vi "Scalar FPGA Personality.vi"() -> ()   [LabVIEW 2018]
uses:
  cRIO RT/TypeDefs/Simple cluster.ctl
  cRIO RT/TypeDefs/Complex cluster.ctl
  <vilib>/rvi/Emulation/niFpgaGetClockAttributes.vi
  <vilib>/rvi/Emulation/niFpgaSctlEmulationGetInTimedLoop.vi
  <vilib>/rvi/Emulation/niFpgaEmulationReportErrorSimple.vi
  <vilib>/rvi/Emulation/niFpgaCriticalErrorInLSC.vi
panel:
  out "Numeric FXP 23/23 out":fxp<+,23,23>
  in  "Numeric FXP 23/23 in":fxp<+,23,23>
  out "Numeric FXP 64/12 out":fxp<+/-,64,12>
  in  "Numeric FXP 64/12 in":fxp<+/-,7,3>
  out "Numeric FXP 7/3 out":fxp<+/-,7,3>
  in  "Numeric FXP 7/3 in":fxp<+/-,64,12>
  in  "Boolean in":bool
  out "Complex cluster out":T1
  in  "Complex cluster in":T1
  out "Simple cluster out":T2
  in  "Simple cluster in":T2
  in  "Numeric FXP 32/16 in":fxp<+/-,32,16>
  in  "Numeric U8 in":u8
  in  "Numeric U16 in":u16
  in  "Numeric U32 in":u32
  in  "Numeric U64 in":u64
  in  "Numeric I8 in":i8
  in  "Numeric I32 in":i32
  in  "Numeric I64 in":i64
  in  "Numeric SGL in":sgl
  in  "Numeric I16 in":i16
  out "Boolean out":bool
  out "Numeric U8 out":u8
  out "Numeric U16 out":u16
  out "Numeric U32 out":u32
  out "Numeric U64 out":u64
  out "Numeric I8 out":i8
  out "Numeric I32 out":i32
  out "Numeric I64 out":i64
  out "Numeric FXP 32/16 out":fxp<+/-,32,16>
  out "Numeric SGL out":sgl
  out "Numeric I16 out":i16
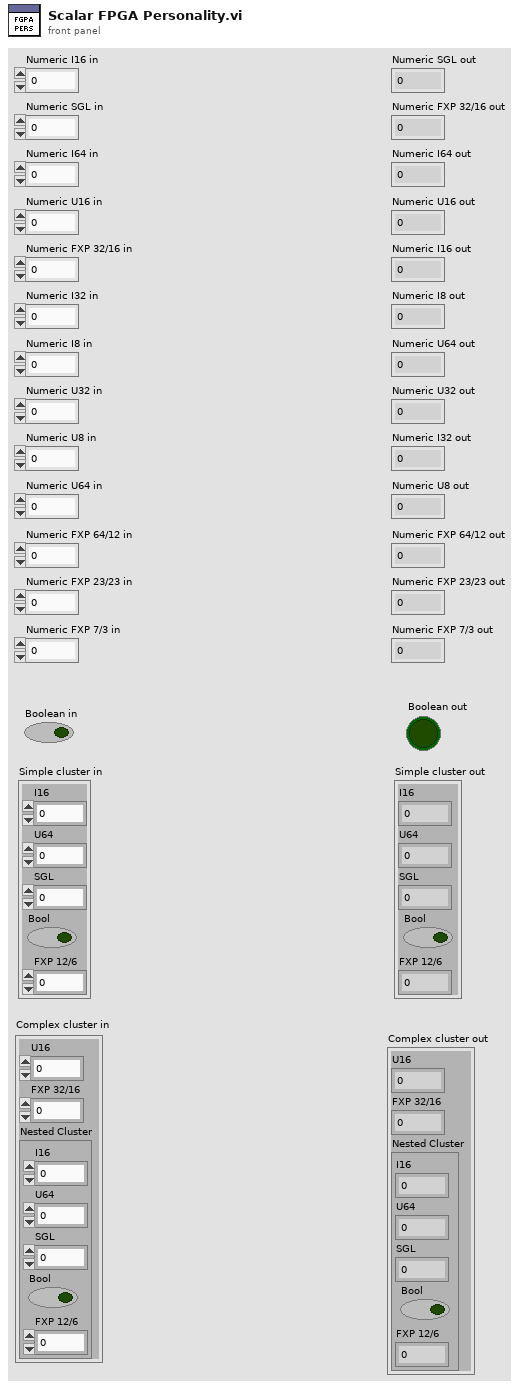
[diagram p1: front panel]
types:
  T1 = typedef "Complex cluster.ctl" = cluster{"U16":u16, "FXP 32/16":fxp<+/-,32,16>, "Nested Cluster":T2}
  T2 = typedef "Simple cluster.ctl" = cluster{"I16":i16, "U64":u64, "SGL":sgl, "Bool":bool, "FXP 12/6":fxp<+/-,12,6>}
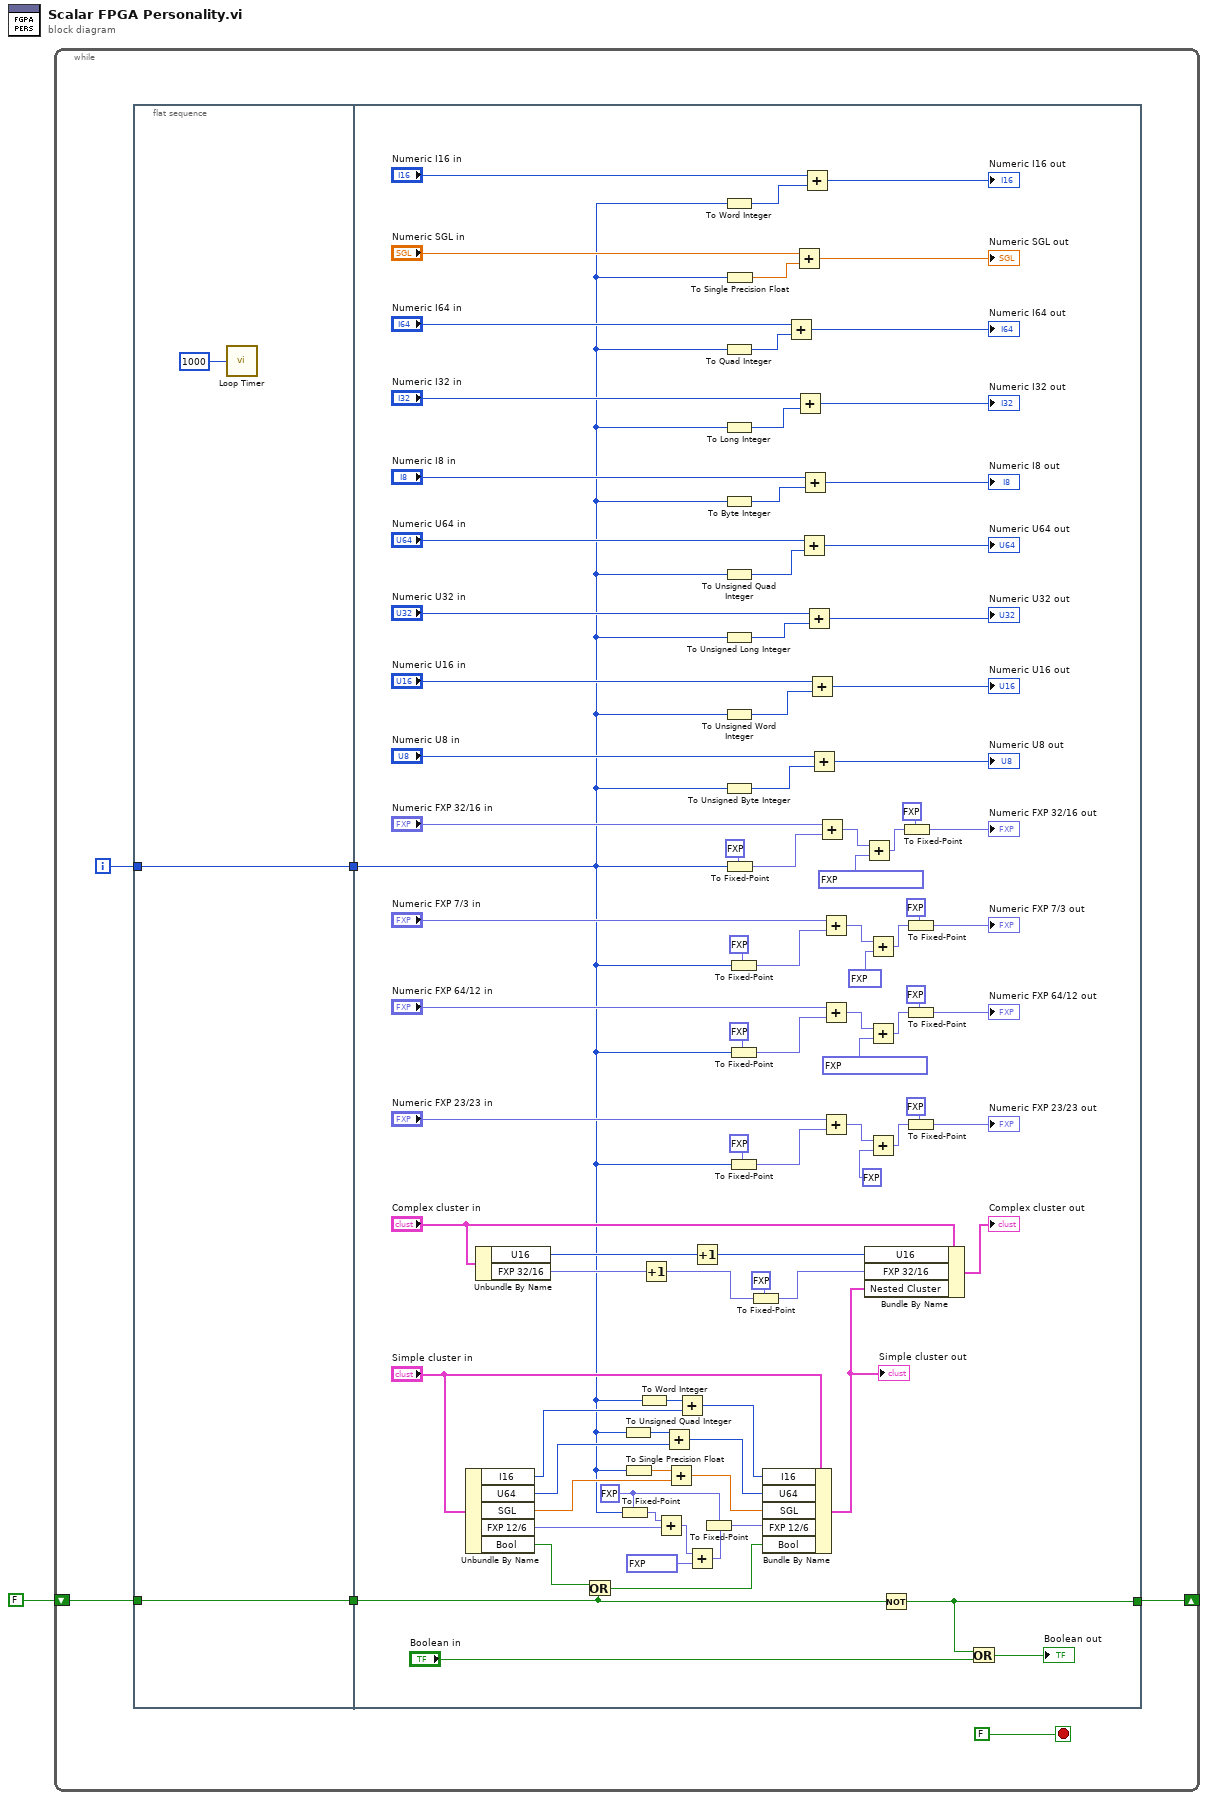
[diagram p0: block diagram]
diagram:
  n1 = while {
    shift-right: [w2] -> _
    shift-left: FALSE -> [w4]
    i -> [w6]
    stop <- FALSE stop-if-true
    n2 = flat-sequence {
      tunnel: w6 -> [w9]
      tunnel: [w9] -> w5
      tunnel: w4 -> [w8]
      tunnel: [w8] -> w3
      tunnel: w5 -> [w11]
      tunnel: w3 -> [w60]
      tunnel: [w38] -> w2
      frame #0 {
        n3 = call "Loop Timer"("Count(mSec)"=u32 1000) -> ()  [unwired: 1 out]
      }
      frame #1 {
        w43 = fxp<+/-,12,6> 0.0 ("FXP 12/6")
        n4 = Unbundle By Name("Simple cluster in") -> ("I16"=w70:i16, "U64"=w69:u64, "SGL"=w65:sgl, "FXP 12/6"=w62:fxp<+/-,12,6>, "Bool"=w59:bool)
        n5 = Unbundle By Name("Complex cluster in") -> ("U16"=w54:u16, "FXP 32/16"=w52:fxp<+/-,32,16>)
        n6 = Or(x=w59, y=w60) -> (x .or. y?=w58:bool)
        n7 = To Fixed-Point(fixed-point type=w43, number=w11) -> (fixed-point=w61:fxp<+/-,12,6>)
        n8 = To Unsigned Quad Integer(1:w11) -> (0:w68:u64)
        n9 = To Single Precision Float(number=w11) -> (single precision float=w64:sgl)
        n10 = To Word Integer(number=w11) -> (16bit integer=w71:i16)
        n11 = Increment(x=w52) -> (x+1=w45:fxp<+/-,33,17>)
        n12 = Add(x=w61, y=w62) -> (x+y=w41:fxp<+/-,13,7>)
        n13 = Add(x=w68, y=w69) -> (x+y=w66:u64)
        n14 = Add(x=w64, y=w65) -> (x+y=w63:sgl)
        n15 = Add(x=w71, y=w70) -> (x+y=w67:i16)
        n16 = Add(x=w41, y=fxp<+/-,12,6> 0.109375 ("FXP 12/6")) -> (x+y=w40:fxp<+/-,14,8>)
        n17 = Increment(x=w54) -> (x+1=w53:u16)
        n18 = To Fixed-Point(fixed-point type=w43, number=w40) -> (fixed-point=w42:fxp<+/-,12,6>)
        n19 = To Word Integer(number=w11) -> (16bit integer=w101:i16)
        n20 = To Quad Integer(1:w11) -> (0:w95:i64)
        n21 = To Long Integer(number=w11) -> (32bit integer=w92:i32)
        n22 = To Byte Integer(number=w11) -> (8bit integer=w89:i8)
        n23 = To Unsigned Quad Integer(1:w11) -> (0:w86:u64)
        n24 = To Unsigned Long Integer(number=w11) -> (unsigned 32bit integer=w83:u32)
        n25 = To Unsigned Word Integer(number=w11) -> (unsigned 16bit integer=w80:u16)
        n26 = To Unsigned Byte Integer(number=w11) -> (unsigned 8bit integer=w77:u8)
        n27 = To Single Precision Float(number=w11) -> (single precision float=w98:sgl)
        n28 = To Fixed-Point(fixed-point type=fxp<+/-,32,16> 0.0, number=w11) -> (fixed-point=w74:fxp<+/-,32,16>)
        n29 = To Fixed-Point(fixed-point type=fxp<+/-,64,12> 0.0, number=w11) -> (fixed-point=w29:fxp<+/-,64,12>)
        n30 = To Fixed-Point(fixed-point type=fxp<+/-,64,12> 0.0, number=w11) -> (fixed-point=w26:fxp<+/-,64,12>)
        n31 = To Fixed-Point(fixed-point type=fxp<+,23,23> 0.0, number=w11) -> (fixed-point=w13:fxp<+,23,23>)
        n32 = To Fixed-Point(fixed-point type=fxp<+/-,32,16> 0.0, number=w45) -> (fixed-point=w44:fxp<+/-,32,16>)
        n33 = Bundle By Name(cluster="Simple cluster in", "I16"=w67, "U64"=w66, "SGL"=w63, "FXP 12/6"=w42, "Bool"=w58) -> (w57:T2)
        "Simple cluster out" <- w57
        n34 = Add(x="Numeric I64 in", y=w95) -> (x+y=→"Numeric I64 out":i64)
        n35 = Add(x="Numeric SGL in", y=w98) -> (x+y=→"Numeric SGL out":sgl)
        n36 = Add(x="Numeric I32 in", y=w92) -> (x+y=→"Numeric I32 out":i32)
        n37 = Add(x="Numeric U64 in", y=w86) -> (x+y=→"Numeric U64 out":u64)
        n38 = Add(x="Numeric I8 in", y=w89) -> (x+y=→"Numeric I8 out":i8)
        n39 = Add(x="Numeric I16 in", y=w101) -> (x+y=→"Numeric I16 out":i16)
        n40 = Add(x="Numeric U32 in", y=w83) -> (x+y=→"Numeric U32 out":u32)
        n41 = Add(x="Numeric U16 in", y=w80) -> (x+y=→"Numeric U16 out":u16)
        n42 = Add(x="Numeric U8 in", y=w77) -> (x+y=→"Numeric U8 out":u8)
        n43 = Add(x="Numeric FXP 32/16 in", y=w74) -> (x+y=w49:fxp<+/-,33,17>)
        n44 = Add(x="Numeric FXP 7/3 in", y=w29) -> (x+y=w33:fxp<+/-,64,13>)
        n45 = Add(x="Numeric FXP 64/12 in", y=w26) -> (x+y=w22:fxp<+/-,64,13>)
        n46 = Add(x="Numeric FXP 23/23 in", y=w13) -> (x+y=w17:fxp<+,24,24>)
        n47 = Add(x=w49, y=fxp<+/-,33,17> 0.111114501953125) -> (x+y=w48:fxp<+/-,34,18>)
        n48 = Bundle By Name(cluster="Complex cluster in", "U16"=w53, "FXP 32/16"=w44, "Nested Cluster"=w57) -> (→"Complex cluster out":T1)
        n49 = Add(x=w33, y=fxp<+/-,7,3> 0.125) -> (x+y=w34:fxp<+/-,64,14>)
        n50 = Add(x=w22, y=fxp<+/-,64,12> 0.111114501953125) -> (x+y=w21:fxp<+/-,64,14>)
        n51 = Add(x=w17, y=fxp<+,23,23> 0.0) -> (x+y=w18:fxp<+,25,25>)
        n52 = Not(x=w60) -> (.not. x?=w38:bool)
        n53 = To Fixed-Point(fixed-point type=fxp<+/-,32,16> 0.0, number=w48) -> (fixed-point=→"Numeric FXP 32/16 out":fxp<+/-,32,16>)
        n54 = To Fixed-Point(fixed-point type=fxp<+/-,7,3> 0.0, number=w34) -> (fixed-point=→"Numeric FXP 7/3 out":fxp<+/-,7,3>)
        n55 = To Fixed-Point(fixed-point type=fxp<+/-,64,12> 0.0, number=w21) -> (fixed-point=→"Numeric FXP 64/12 out":fxp<+/-,64,12>)
        n56 = To Fixed-Point(fixed-point type=fxp<+/-,23,23> 0.0, number=w18) -> (fixed-point=→"Numeric FXP 23/23 out":fxp<+/-,23,23>)
        n57 = Or(x=w38, y="Boolean in") -> (x .or. y?=→"Boolean out":bool)
      }
    }
  }
